vi "Internal Project Home.vi"(4 "Function":enum16{"Read", "Write"}(ring), 5 "Error In":errorcluster, 8 "Top-Level VI Path":path) -> (0 "Error Out":errorcluster, 3 "Internal Home Path":path)   [LabVIEW 2014, in "Path Utilities.lvlib"]
uses:
  Path Utilities.lvlib
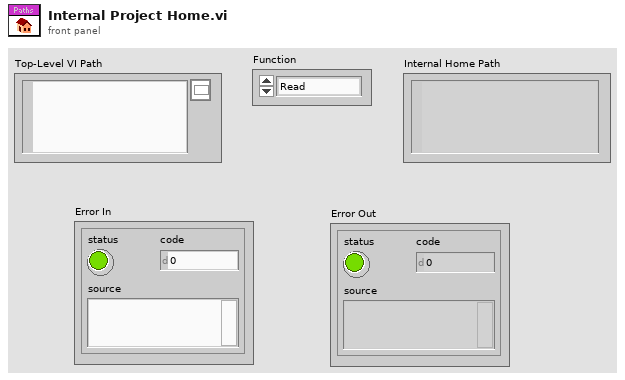
[diagram p1: front panel]
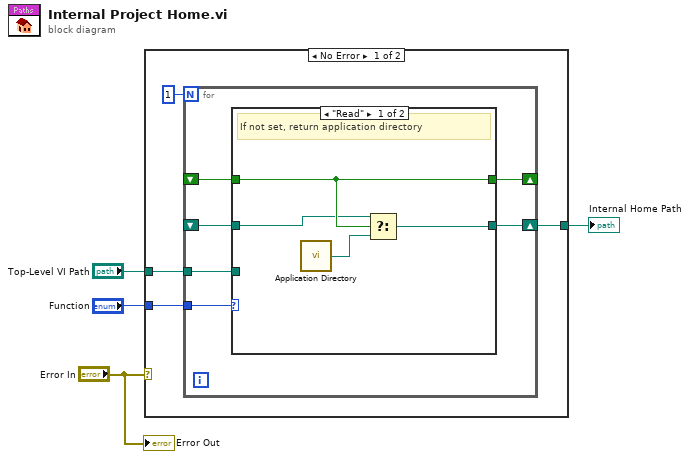
[diagram p0: block diagram]
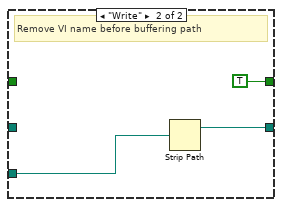
[diagram p2: hidden frame]
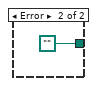
[diagram p3: hidden frame]
diagram:
  n1 = case shown="No Error" "Error In" {
    tunnel: "Function" -> [w7 _]
    tunnel: "Top-Level VI Path" -> [w6 _]
    tunnel: [w5 path ""] -> w2
    frame No Error {
      n2 = for {
        N: 1 -> [_]
        shift-right: [w13] -> w5
        shift-left: _ -> [w14]
        tunnel: w7 -> [w12]
        tunnel: w6 -> [w11]
        shift-right: [w9] -> _
        shift-left: _ -> [w10]
        n3 = case shown="\"Read\"" w12 {
          tunnel: w14 -> [w16 _]
          tunnel: [w17 w20] -> w13
          tunnel: w11 -> [_ w21]
          tunnel: w10 -> [w18 _]
          tunnel: [w18 TRUE] -> w9
          frame "Read" {
            # "If not set, return application directory"
            n4 = call <vilib>:"Application Directory.vi"() -> ("Application Directory"=w15:path)
            n5 = Select(t=w16, s=w18, f=w15) -> (s? t:f=w17:path)
          }
          frame "Write" {
            # "Remove VI name before buffering path"
            n6 = Strip Path(path=w21) -> (stripped path=w20:path)  [unwired: 1 out]
          }
        }
      }
    }
    frame Error {
    }
  }
  "Internal Home Path" <- w2
  "Error Out" <- "Error In"
